vi "Get Info.vi"(8 "error in (no error)":errorcluster, 11 "Reader in":refnum<class "Reader.lvclass">) -> (0 "error out":errorcluster, 1 "Number of Frames":u64, 2 "Size":T1, 3 "Reader":refnum<class "Reader.lvclass">, 4 "FPS":dbl)   [LabVIEW 2020, in "video_io.lvlib" / "Reader.lvclass"]
uses:
  Reader ARGB/Reader.lvclass
  Reader ARGB/Reader.lvclass/Reader.ctl
  common/common.lvlib
  common/Image Size (Integer).ctl
  common/bin/gartoolkit_32-1.dll
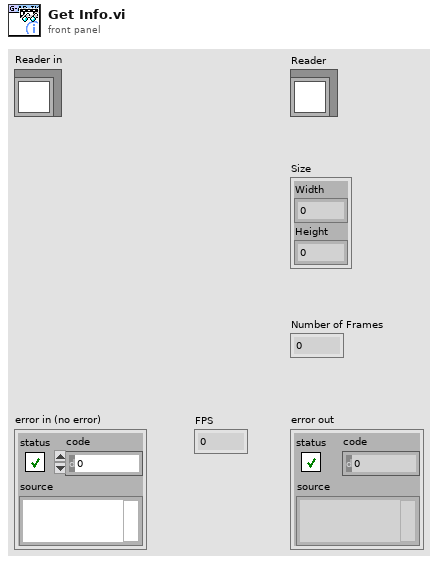
[diagram p1: front panel]
types:
  T1 = typedef "common.lvlib/Image Size (Integer).ctl" = cluster{"Width":u16, "Height":u16}
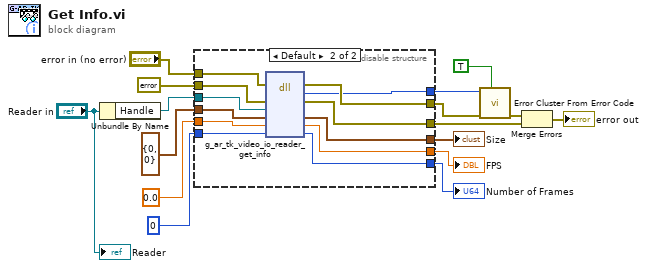
[diagram p0: block diagram]
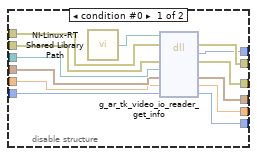
[diagram p2: hidden frame]
diagram:
  n1 = Unbundle By Name("Reader in") -> ("Handle"=w8:refnum<data-value>)
  n2 = disable-structure shown="Default" {
    disable-tunnel: "error in (no error)" -> [w28 w41]
    disable-tunnel: errorcluster {"status"=FALSE, "code"=0, "source"=""} ("error constant") -> [w27 w40]
    disable-tunnel: w8 -> [w26 w39]
    disable-tunnel: [w19 w38] -> w13
    disable-tunnel: [w18 w37] -> w12
    disable-tunnel: [w17 w36] -> w10
    disable-tunnel: T1 {"Width"=0, "Height"=0} ("Image Size") -> [w25 w35]
    disable-tunnel: [w20 w34] -> w5
    disable-tunnel: [w22 w33] -> w4
    disable-tunnel: [w21 w32] -> w3
    disable-tunnel: 0.0 ("fps") -> [w24 w31]
    disable-tunnel: u64 0 ("n_frames") -> [w23 w30]
    frame condition #0 {
      n3 = call "NI-Linux-RT Shared Library Path.vi"() -> ("Path"=w29:path)
      n4 = dll-call lib="?" fn="g_ar_tk_video_io_reader_get_info" ("g_ar_toolkit.*.*:g_ar_tk_capture_context_create")(path in=w29, error in=w28, "error_cluster"=w27, "Handle"=w26, "size"=w25, "fps"=w24, "n_frames"=w23) -> (error out=w19:errorcluster, "return type"=w18:i32, "error_cluster"=w17:errorcluster, "size"=w20:T1, "fps"=w22:dbl, "n_frames"=w21:u64)  [unwired: 2 in, 1 out]
    }
    frame condition #1 (active) {
      n5 = dll-call lib="C:/serenial/lib/g-augmented-reality-toolkit/LabVIEW/common/bin/gartoolkit_*-1.*" fn="g_ar_tk_video_io_reader_get_info" ("g_ar_toolkit.*.*:g_ar_tk_capture_context_create")(error in=w41, "error_cluster"=w40, "Handle"=w39, "size"=w35, "fps"=w31, "n_frames"=w30) -> (error out=w38:errorcluster, "return type"=w37:i32, "error_cluster"=w36:errorcluster, "size"=w34:T1, "fps"=w33:dbl, "n_frames"=w32:u64)  [unwired: 3 in, 1 out]
    }
  }
  "Size" <- w5
  "FPS" <- w4
  "Number of Frames" <- w3
  n6 = call <vilib>:"Error Cluster From Error Code.vi"("show call chain? (False)"=TRUE, "error in (no error)"=w13, "error code (0)"=w12) -> ("error out"=w16:errorcluster)  [unwired: 6 in]
  n7 = Merge Errors(w16, w10) -> (→"error out":errorcluster)
  "Reader" <- "Reader in"
